vi "Launcher.vi"() -> ()   [LabVIEW 2019]
uses:
  UI Actor/UI Actor.lvclass
  C:/Program Files (x86)/National Instruments/LabVIEW 2019/vi.lib/ActorFramework/Actor/Actor.lvclass
  UI Actor/UI Actor.lvclass/UI Actor.ctl
  UI Actor/Write Monedas.vi
  UI Actor/Write Productos.vi
  UI Actor/Write Mensajes.vi
  <vilib>/ActorFramework/Actor/Actor.lvclass
panel:
  in  "Mensajes":enum16{"Ingles", "Español"}(ring)
  in  "Productos":enum16{"Refrescos y Papas", "Cafe"}(ring)
  in  "Monedas":enum16{"MXN", "USD"}(ring)
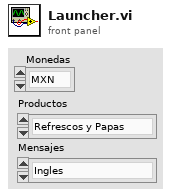
[diagram p1: front panel]
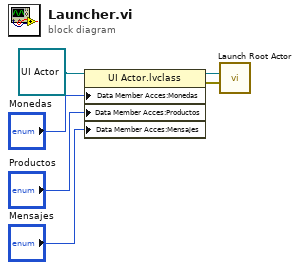
[diagram p0: block diagram]
diagram:
  n1 = property class="UI Actor.lvclass"(reference=refnum<class "UI Actor.lvclass"> refnum ("UI Actor.lvlib:UI Actor.lvclass"), "Data Member Acces:Monedas"="Monedas", "Data Member Acces:Productos"="Productos", "Data Member Acces:Mensajes"="Mensajes") -> (reference out=w4:refnum<class "UI Actor.lvclass">, error out=w3:errorcluster)  [unwired: 1 in]
  n2 = call <vilib>:"Launch Root Actor.vi"("error in (no error)"=w3, "Actor"=w4) -> ()  [unwired: 8 in, 2 out]
